vi "Reset Errno Value for Calling Thread.vi"(8 "error in (no error)":errorcluster) -> (0 "error out":errorcluster)   [LabVIEW 2013, in "Linux Errno.lvlib"]
doc: "This VI resets the value of the errno variable for the calling thread to zero. This is useful in cases where a function only sets the errno variable in the event of an error, and any previous value of errno from a previous function is preserved."
uses:
  Linux Errno.lvlib
panel:
  out "value":i32
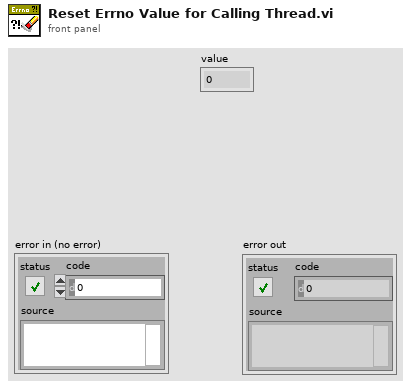
[diagram p1: front panel]
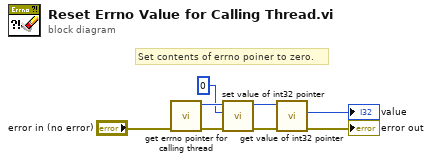
[diagram p0: block diagram]
diagram:
  # "Set contents of errno poiner to zero."
  n1 = call "get errno pointer for calling thread.vi"("error in (no error)"="error in (no error)") -> ("error out"=w7:errorcluster, "errno pointer"=w6:u64)  [unwired: 9 in]
  n2 = call "set value of int32 pointer.vi"("error in (no error)"=w7, "value (0)"=0, "pointer in"=w6) -> ("error out"=w5:errorcluster, "pointer out"=w3:u64)  [unwired: 7 in]
  n3 = call "get value of int32 pointer.vi"("error in (no error)"=w5, "pointer in"=w3) -> ("error out"=→"error out":errorcluster, "value"=→"value":i32)  [unwired: 7 in, 1 out]
